vi "Instances string to array.vi"(1 "String":string="1, 2, 2, 3, 4, 5,   7, 6 and 9") -> (0 "Array":string[](array[string]))   [LabVIEW 2015]
uses:
  <vilib>/regexp/Match Regular Expression.xnode
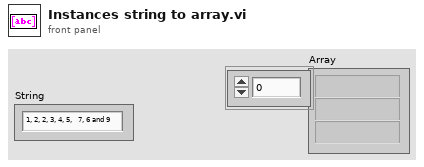
[diagram p1: front panel]
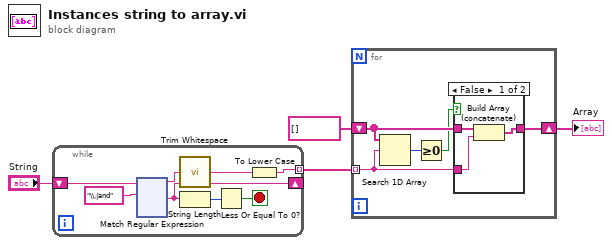
[diagram p0: block diagram]
diagram:
  n1 = while {
    tunnel: [w5] -> w3 mode=indexing
    shift-right: [w10] -> _
    shift-left: "String" -> [w7]
    stop <- w8 stop-if-true
    n2 = xnode "Match Regular Expression"("input string"=w7, "regular expression"="\\,|and" ("search string/char (-)")) -> ("before match"=w11:string, "after match"=w10:string)  [unwired: 4 in, 3 out]
    n3 = call <vilib>:"Trim Whitespace.vi"("string"=w11) -> ("trimmed string"=w6:string)  [unwired: 1 in]
    n4 = String Length(string=w10) -> (length=w9:i32)
    n5 = Less Or Equal To 0?(x=w9) -> (x <= 0?=w8:bool)
    n6 = To Lower Case(string=w6) -> (all lower case string=w5:string)
  }
  n7 = for {
    tunnel: w3 -> [w130] mode=indexing
    shift-right: [w129] -> w1
    shift-left: string[] [] -> [w131]
    n8 = Search 1D Array(1D array=w131, element=w130) -> (index of element=w128:i32)  [unwired: 1 in]
    n9 = Greater Or Equal To 0?(x=w128) -> (x >= 0?=w127:bool)
    n10 = case shown="False" w127 {
      tunnel: w131 -> [w134 w135]
      tunnel: w130 -> [w133 _]
      tunnel: [w132 w135] -> w129
      frame False {
        n11 = Build Array (concatenate)(w134, w133) -> (w132:string[])
      }
      frame True {
      }
    }
  }
  "Array" <- w1
